vi "Get Motor Angle.vi"(1 "Encoder Resolution":i32, 2 "Encoder Value":i32) -> (0 "Motor Angle":dbl)   [LabVIEW 2019]
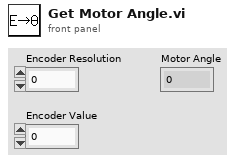
[diagram p1: front panel]
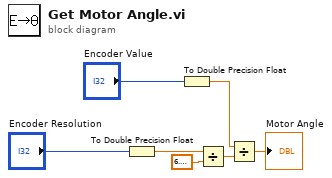
[diagram p0: block diagram]
diagram:
  n1 = To Double Precision Float(number="Encoder Resolution") -> (double precision float=w3:dbl)
  n2 = To Double Precision Float(number="Encoder Value") -> (double precision float=w1:dbl)
  n3 = Divide(x=w3, y=6.283185307179586) -> (x/y=w5:dbl)
  n4 = Divide(x=w1, y=w5) -> (x/y=→"Motor Angle":dbl)
